vi "Construct_multipart_message_notresponse.vi"(0 "command":T1=enum."configure_rf", 5 "parameters (JSON)":string="{\"invalid\":1}", 9 "data in":string, 11 "error in (no error)":errorcluster) -> (3 "command_str":string="invalid_command", 4 "Multipart message":string[](array[string]), 14 "Debug info":string, 15 "error out":errorcluster)   [LabVIEW 2019, in "mmW_commands.lvlib"]
uses:
  TypeDefs/commands.ctl
  mmW_commands.lvlib
panel:
  out "type (none)":string="none"
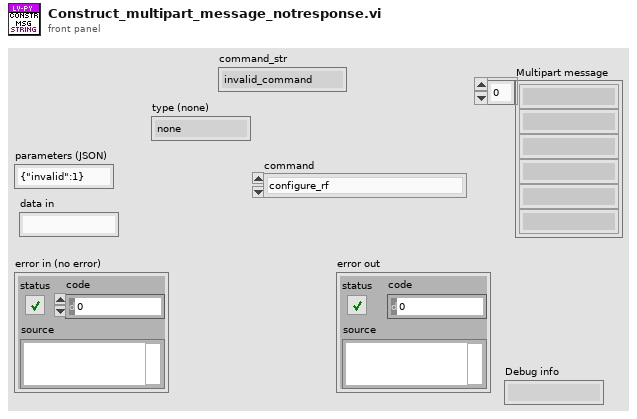
[diagram p1: front panel]
types:
  T1 = typedef "mmW_commands.lvlib/commands.ctl" = enum16{"configure_fs", "configure_rf", "configure_trigger", "equalization_enable", "equalization_start", "lo_sync_enable", "equalization_stop", "get_instrument_status", "get_versions", "initialize_hw", "pop_rx", "set_log_level", "Shutdown", "start", "start_instrument_app", "stop", "trans", "transceive", "trigger_burst", "trigger_sync_enable", "Write TX", "resp_generic", "resp_waveform", "send_trigger", "fetch", "transceive2"}
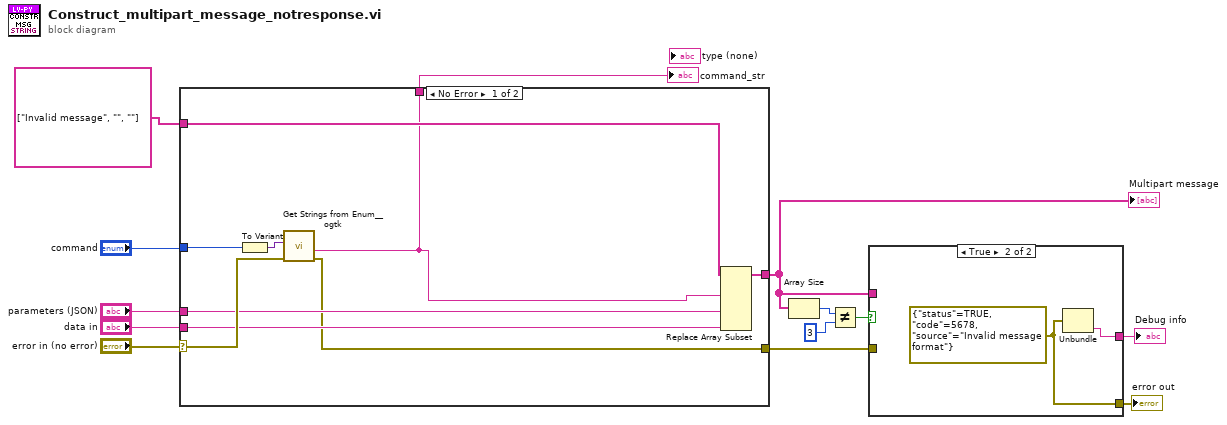
[diagram p0: block diagram]
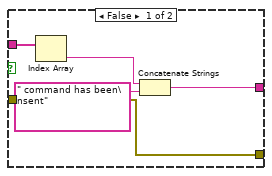
[diagram p2: hidden frame]
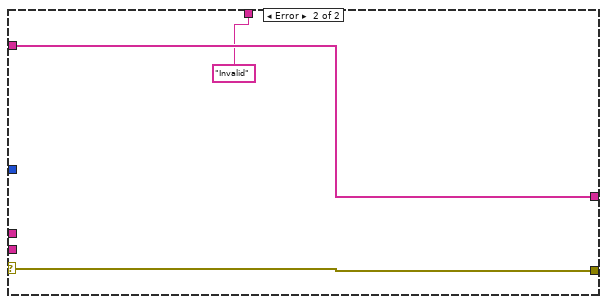
[diagram p3: hidden frame]
diagram:
  n1 = case shown="No Error" "error in (no error)" {
    selector: "error in (no error)" -> [w18 w24]
    tunnel: "parameters (JSON)" -> [w16 _]
    tunnel: [w15 w24] -> w6
    tunnel: [w22 w25] -> w5
    tunnel: string[] ["Invalid message", "", ""] -> [w21 w25]
    tunnel: "command" -> [w19 _]
    tunnel: [w14 "Invalid" ("String Value")] -> w2
    tunnel: "data in" -> [w17 _]
    frame No Error {
      n2 = To Variant(anything=w19) -> (Variant=w20:variant)
      n3 = call <userlib>:"Get Strings from Enum__ogtk.vi"("error in (no error)"=w18, "Enum"=w20) -> ("error out"=w15:errorcluster, "String Value"=w14:string)  [unwired: 6 in, 2 out]
      n4 = Replace Array Subset(array=w21, new element #1=w14, new element #2=w16, new element #3=w17) -> (w22:string[])  [unwired: 3 in]
    }
    frame Error {
    }
  }
  "Multipart message" <- w5
  "command_str" <- w2
  n5 = Array Size(array=w5) -> (size(s)=w10:i32)
  n6 = Not Equal?(x=w10, y=3) -> (x != y?=w8:bool)
  n7 = case shown="True" w8 {
    tunnel: [w30 w32] -> w7
    tunnel: w6 -> [w30 _]
    tunnel: w5 -> [w29 _]
    tunnel: [w26 w31] -> w4
    frame False {
      n8 = Index Array(array=w29) -> (element=w28:string)  [unwired: 1 in]
      n9 = Concatenate Strings(w28, " command has been\nsent" ("string")) -> (w26:string)
    }
    frame True {
      w32 = errorcluster {"status"=TRUE, "code"=5678, "source"="Invalid message format"} ("s? t:f")
      n10 = Unbundle(w32) -> ("source"=w31:string)  [unwired: 2 out]
    }
  }
  "error out" <- w7
  "Debug info" <- w4
